vi "Client CR.vi"() -> ()   [LabVIEW 2021]
uses:
  Master CR/Examples/PM3112/enums/main_prog_state.ctl
  Master CR/Examples/PM3112/enums/init_state.ctl
  WebSockets/WebSocket Client CR/WebSocket Client CR.lvclass
  Master CR/Param/TCP Param/TCP Param.lvclass
  D:/my_projects/projects/Algorithms/Labview/21/Master CR/Param/Param.lvclass
  WebSockets/WebSocket Client CR/WebSocket Client CR.lvclass/WebSocket Client CR.ctl
  Master CR/Param/Param.lvclass/Param.ctl
  Master CR/Param/TCP Param/TCP Param.lvclass/TCP Param.ctl
  <vilib>/Platform/TimedLoop/XDataNode/timing_clust.ctl
  <vilib>/Platform/TimedLoop/XDataNode/nitl_modes.ctl
  <vilib>/Platform/TimedLoop/XDataNode/wakeup.ctl
  Master CR/Examples/PM3112/enums/close_state.ctl
  <vilib>/Platform/TimedLoop/XDataNode/XDataNode.xnode
  Modbus_v121c/Data Model/Device Data Model.lvclass
  <vilib>/Platform/TimedLoop/XDataNode/XDNodeRunTimeDep.lvlib
  Master CR/Examples/PM3112/enums/Param_MB test.lvlib
  Master CR/Param/Param.lvclass
panel:
  in  "Send String Data":string[](array[string])
  out "String Data":string[](array[string])
  in  "Write":bool
  in  "Read":bool
  out "connects":bool[](array[boolean])
  out "Binary Data":u8[][](array[numeric])
  in  "Send Binary Data":u16[][](array[numeric])
  out "comm error":errorcluster
  out "initialise error":errorcluster
  in  "EP_on":bool
  in  "tick":i64=100 caption="Время цикла основной программы" min=5 max=500 step=1
  in  "stop":bool
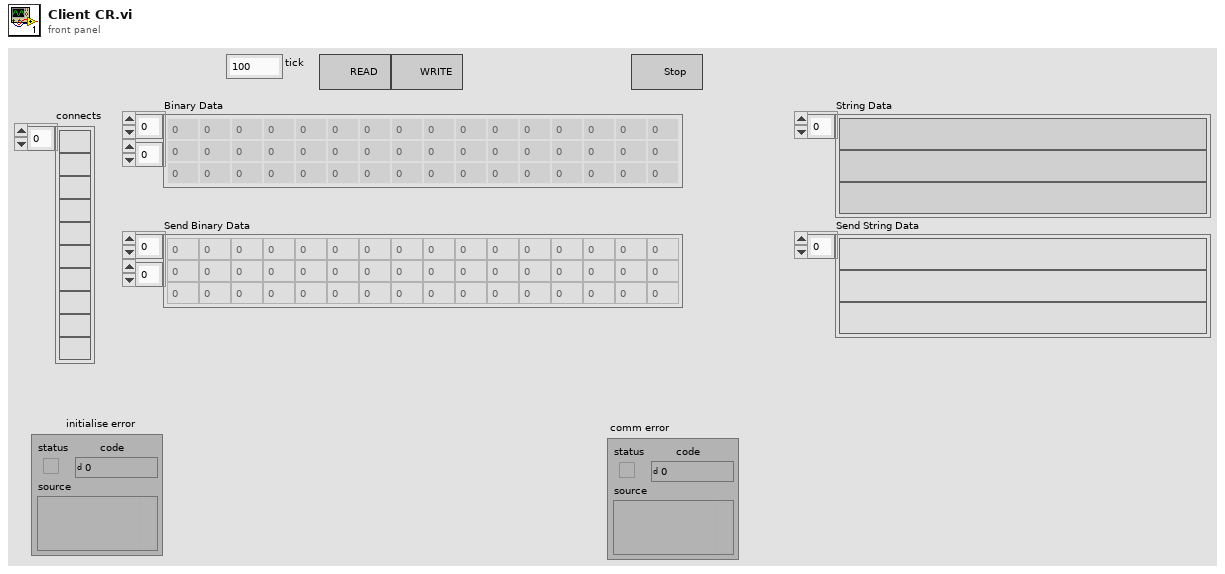
[diagram p1: front panel]
types:
  T1 = cluster{"conn_timeout":i32, "reconn_timeout":i32, "N attempt max":i32, "t_reset_TTL":i32, "write_timeout":i32, "read_timeout":i32, "period":i32}[]
  T2 = cluster{"Remote IP Address":string, "Remote Port":u16}[]
  T3 = typedef "Param_MB test.lvlib/init_state.ctl" = enum16{"Init Data", "Init TMPs", "Init system DB", "Init data DB", "Read Enums", "Init arrays", "Init KFM", "Init Param", "Init AI param", "Init DI param", "Init AO param", "Init DO param", "Init ALR param", "Init save progs", "Read OPC param", "Init Shared Variables", "Init regulators", "Init heaters", "Init Y defs", "Exit"}
  T4 = typedef "Param_MB test.lvlib/main_prog_state.ctl" = enum16{"Read_AI_Param", "Read_DI_Param", "Read_AO_Param", "Read_DO_Param", "Read_ALR_ON_OFF", "Read_ALR_Param", "Read_Param", "Read_REG_Param", "Timers", "AI", "DI", "SendAItoScada", "SendDItoScada", "Alarms", "SendAItoDB", "SendDItoDB", "SendALRtoDB", "Messages", "Controls", "Control HT1", "QN_control", "QN", "QN_state", "Control EB3", "Outputs", "Exit"}
  T5 = cluster{"KFM":string[], "PAR":string[], "AI":string[], "DI":string[], "DI_fast":string[], "AO":string[], "Regs":string[], "DO":string[], "ALR":string[], "System":string[]}
  T6 = cluster{"Enums":cluster{"KFM":string[], "PAR":string[], "AI":string[], "DI":string[], "DI_fast":string[], "AO":string[], "Regs":string[], "DO":string[], "ALR":string[], "System":string[]}, "WSs":refnum<class "WebSocket Client CR.lvclass">[]}
  T7 = cluster{"current time":timestamp, "Timer_1s":bool, "Timer_10s":bool, "Timer_1day":bool}
  T8 = typedef "XDNodeRunTimeDep.lvlib/timing_clust.ctl" = cluster{"Expected End [f-1]":u64, "Actual End [f-1]":u64, "Finished Late? [f-1]":bool, "Expected End [i-1]":u64, "Actual End [i-1]":u64, "Finished Late? [i-1]":bool, "Expected Start [i]":u64, "Actual Start [i]":u64, "Expected Start [f]":u64, "Actual Start [f]":u64, "Source Name":string, "Structure Name":string, "Period":i64, "Deadline":i64, "Offset":i64, "Start":i64, "Priority":i32, "Timeout":i32, "Mode":T9, "Wakeup Reason":T10, "Error":errorcluster, "Source Type":string, "Secondary Source Type":string, "Global End Time":u64, "Global Start Time":u64, "Frame Duration":u64, "Iteration Duration":u64, "Assigned CPU":i32, "I/O Scan Engine Mode":u32}
  T9 = typedef "XDNodeRunTimeDep.lvlib/nitl_modes.ctl" = enum32{"No Change", "Process missed periods, maintain original phase", "Discard missed periods, maintain original phase", "Process missed periods, ignore original phase", "Discard missed periods, ignore original phase"}
  T10 = typedef "XDNodeRunTimeDep.lvlib/wakeup.ctl" = enum32{"Normal", "Aborted", "Asynchronous wakeup", "Timing source error", "Timed loop error", "Timeout"}
  T11 = typedef "Param_MB test.lvlib/close_state.ctl" = enum16{"QN_state notifier", "QN_control_queue", "ALR notifires", "ALR", "DO notifires", "DO", "AO notifires", "AO", "DI notifres", "DI", "AI notifires", "AI", "OPC", "Param", "SaveMessageProg", "KFM DadaRef", "KFM Registers", "KFM StatusRef", "Exit"}
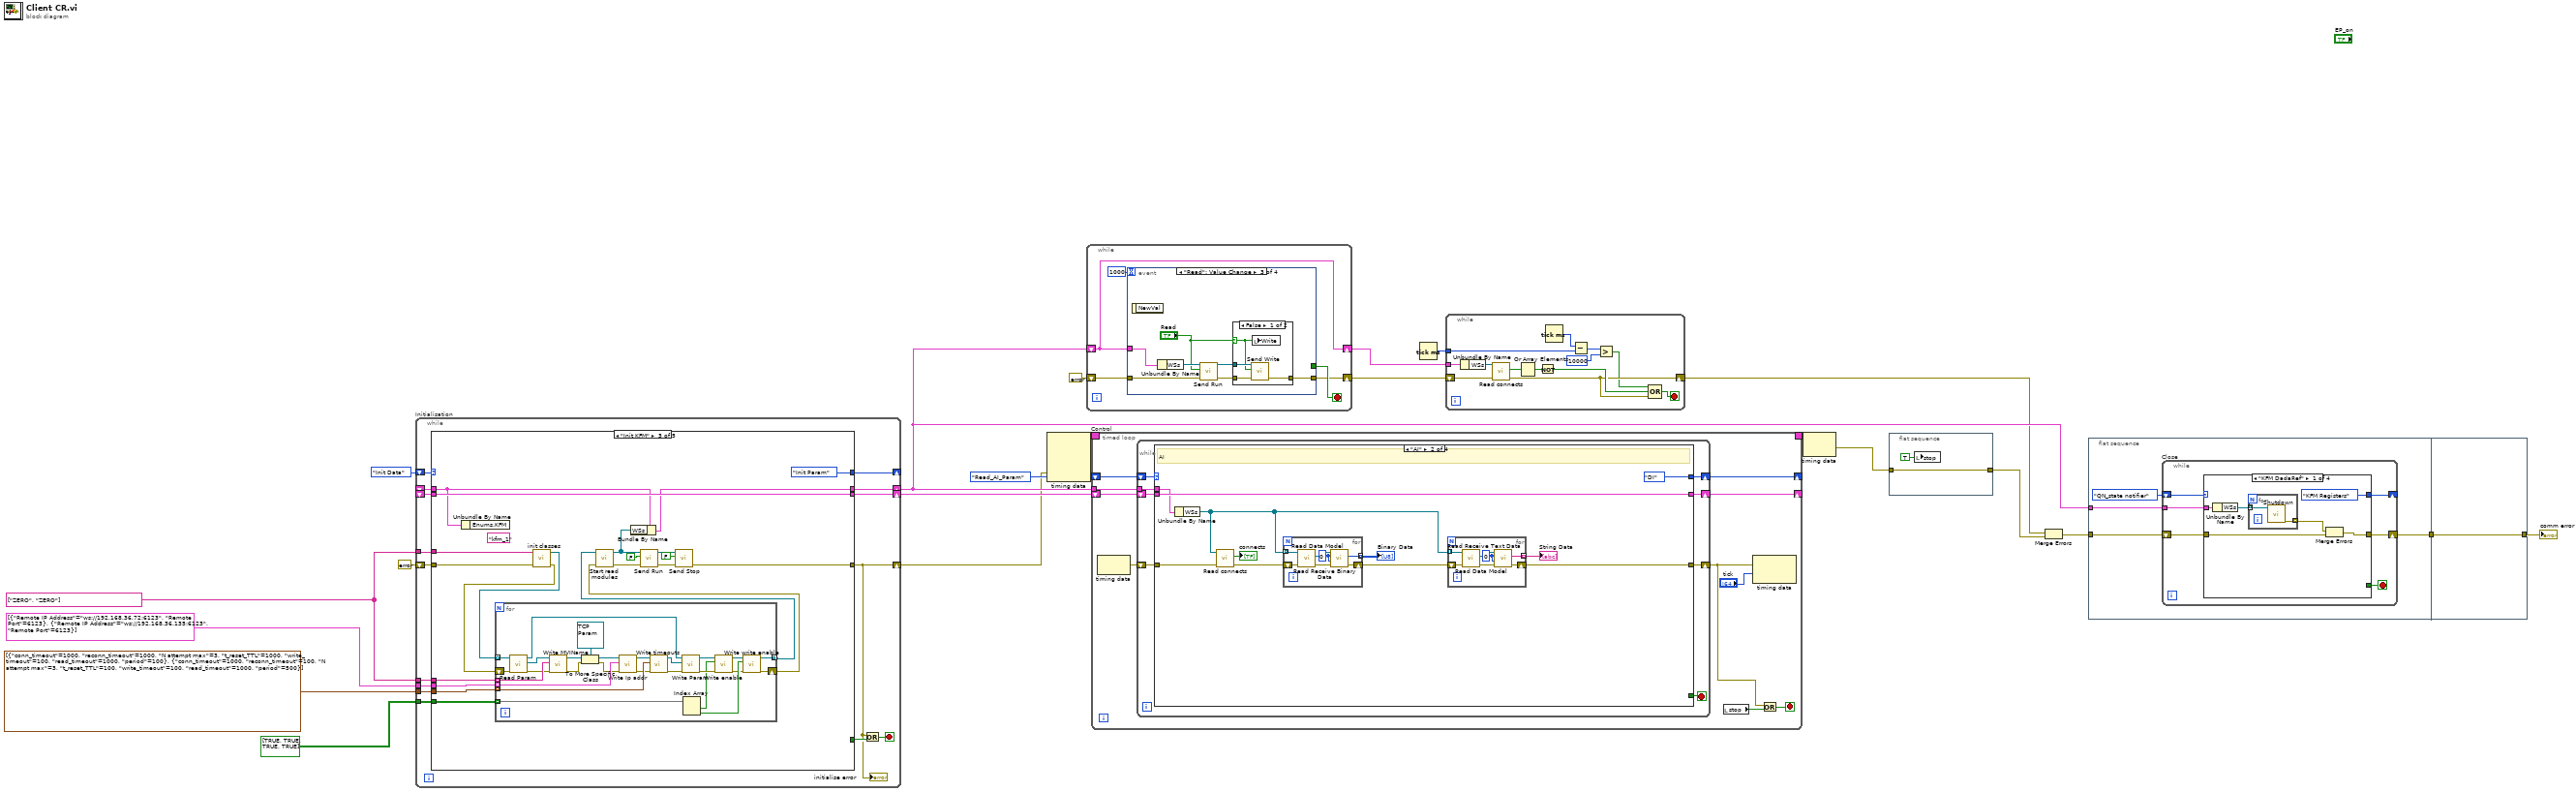
[diagram p0: block diagram]
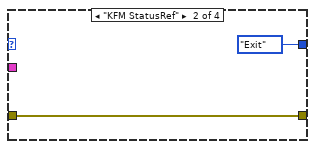
[diagram p2: hidden frame]
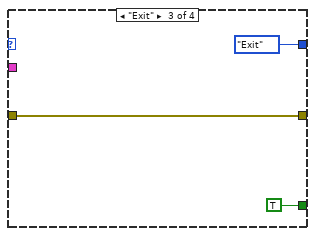
[diagram p3: hidden frame]
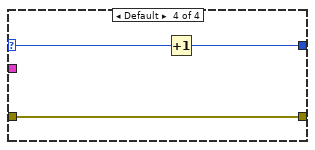
[diagram p4: hidden frame]
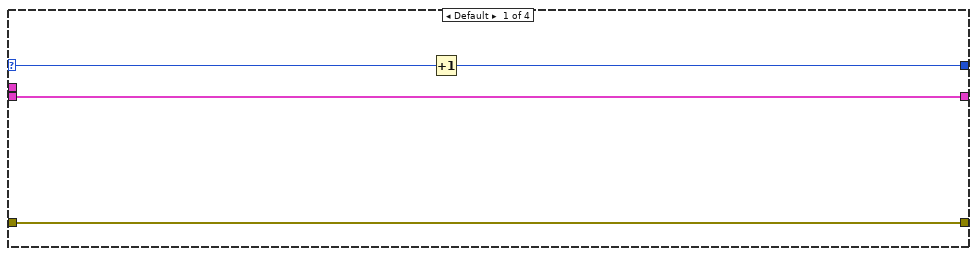
[diagram p5: hidden frame]
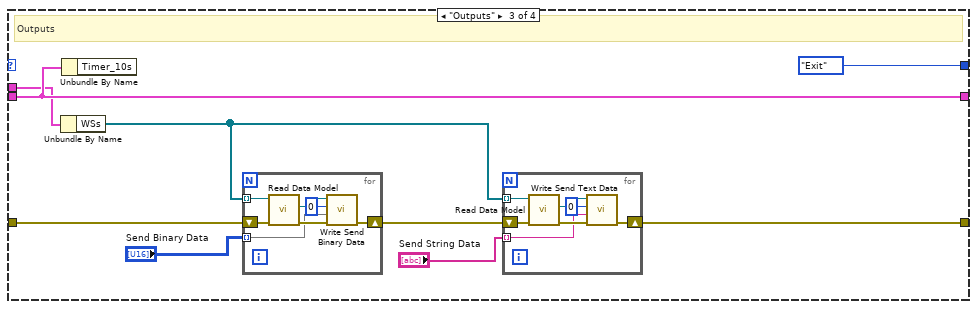
[diagram p6: hidden frame]
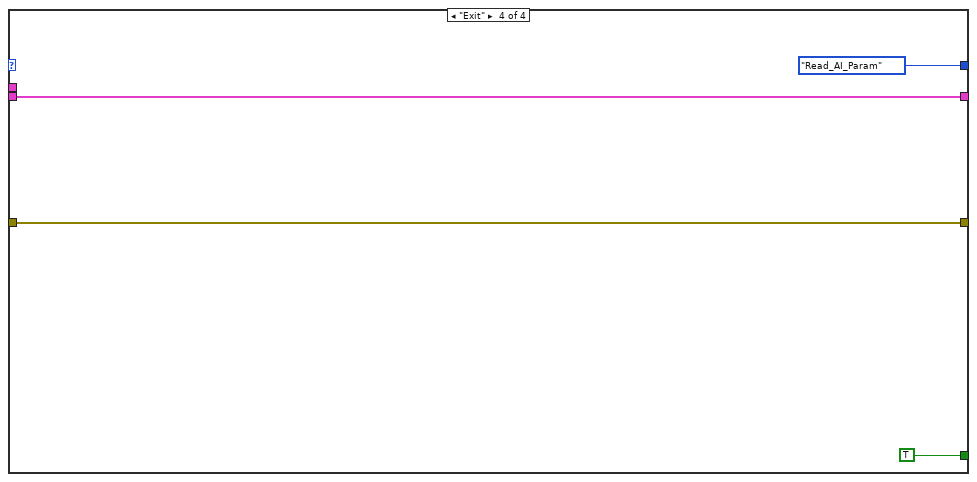
[diagram p7: hidden frame]
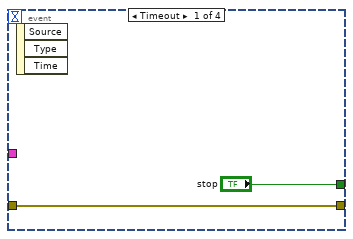
[diagram p8: hidden frame]
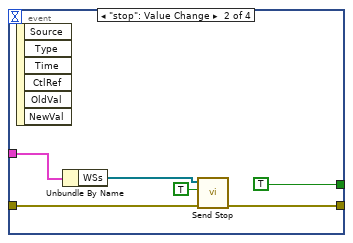
[diagram p9: hidden frame]
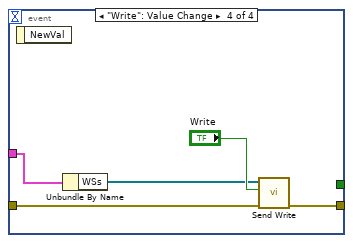
[diagram p11: hidden frame]
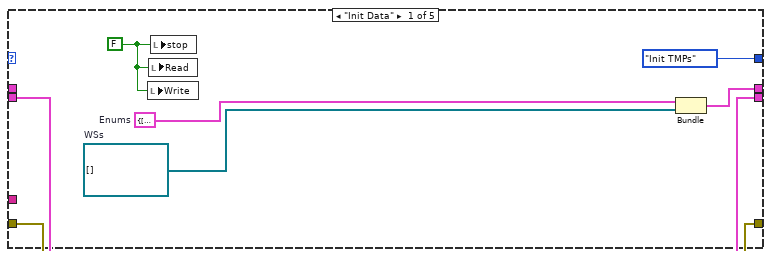
[diagram p12: hidden frame]
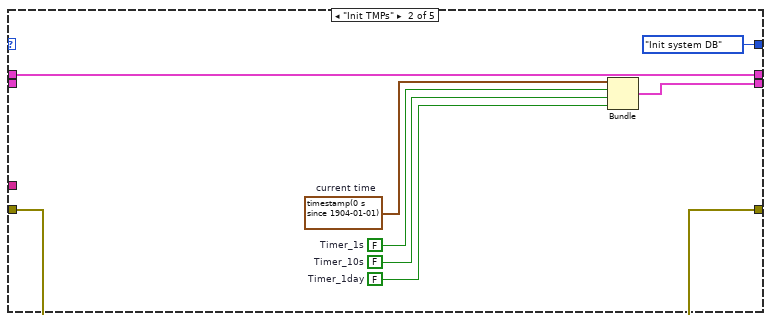
[diagram p13: hidden frame]
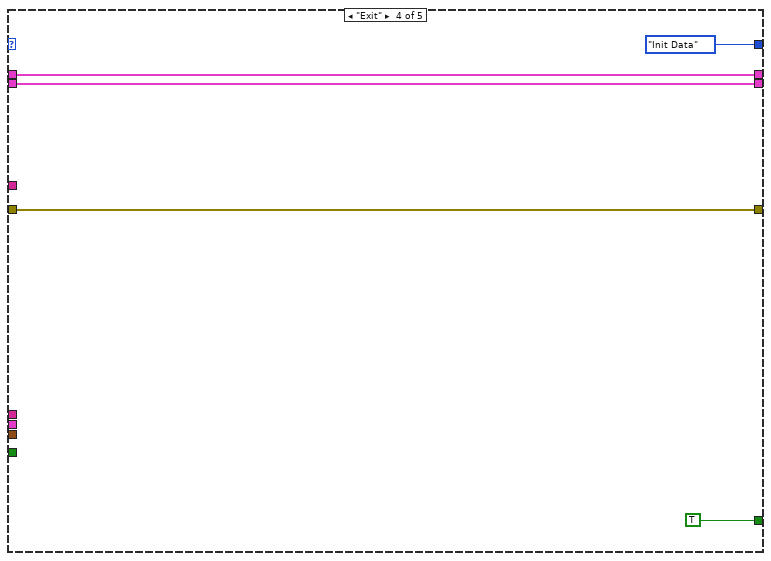
[diagram p14: hidden frame]
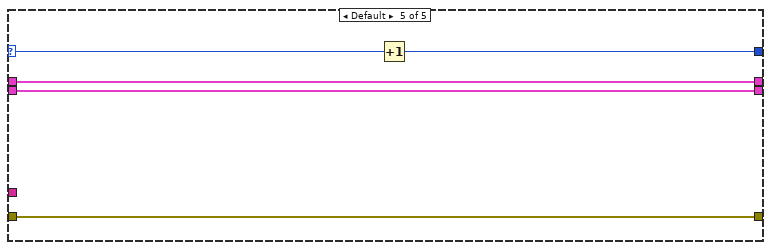
[diagram p15: hidden frame]
diagram:
  w8 = string[] ["ZERO", "ZERO"] ("MVIName")
  n1 = while "Initialisation" {
    shift-right: [w28] -> w7
    shift-left: errorcluster {"status"=FALSE, "code"=0, "source"=""} ("error out") -> [w34]
    shift-right: [w37] -> w13
    shift-left: _ -> [w35]
    shift-right: [w33] -> _
    shift-left: init_state."Init Data" -> [w36]
    shift-right: [w30] -> w16
    shift-left: _ -> [w29]
    tunnel: w8 -> [w27]
    tunnel: T2 [{"Remote IP Address"="ws://192.168.36.72:6123", "Remote Port"=6123}, {"Remote IP Address"="ws://192.168.36.135:6123", "Remote Port"=6123}] ("IP Address") -> [w26]
    tunnel: T1 [{"conn_timeout"=1000, "reconn_timeout"=1000, "N attempt max"=3, "t_reset_TTL"=1000, "write_timeout"=100, "read_timeout"=1000, "period"=100}, {"conn_timeout"=1000, "reconn_timeout"=100, "N attempt max"=3, "t_reset_TTL"=100, "write_timeout"=100, "read_timeout"=1000, "period"=500}] ("timeouts") -> [w25]
    tunnel: bool[][] [[TRUE, TRUE], [TRUE, TRUE]] ("enable") -> [w24]
    tunnel: w8 -> [w23]
    stop <- w31 stop-if-true
    # "Initialisation"
    n2 = case shown="\"Init KFM\"" w36 {
      tunnel: [w42 w51 w53 w102 w105] -> w28
      selector: w36 -> [_ _ _ _ w108]
      tunnel: [w43 w50 w54 w103 w106] -> w37
      tunnel: w35 -> [_ w50 w71 w103 w106]
      tunnel: w34 -> [w42 w51 w70 w102 w105]
      tunnel: [init_state."Init TMPs" init_state."Init system DB" init_state."Init Param" init_state."Init Data" w107] -> w33
      tunnel: [_ _ _ TRUE _] -> w32
      tunnel: [w40 w49 w72 w100 w109] -> w30
      tunnel: w29 -> [w40 _ w72 w100 w109]
      tunnel: w27 -> [_ _ w65 _ _]
      tunnel: w26 -> [_ _ w64 _ _]
      tunnel: w25 -> [_ _ w63 _ _]
      tunnel: w24 -> [_ _ w62 _ _]
      tunnel: w23 -> [_ _ w61 _ _]
      frame "Init Data" {
        w38 = refnum<class "WebSocket Client CR.lvclass">[] []  # WSs
        w39 = FALSE ("stop")
        w41 = T5 {"KFM"=[], "PAR"=[], "AI"=[], "DI"=[], "DI_fast"=[], "AO"=[], "Regs"=[], "DO"=[], "ALR"=[], "System"=[]}  # Enums
        n3 = local write "Write"(w39) -> ()
        n4 = local write "Read"(w39) -> ()
        n5 = local write "stop"(w39) -> ()
        n6 = Bundle("Enums"=w41, "WSs"=w38) -> (w43:T6)  [unwired: 1 in]
      }
      frame "Init TMPs" {
        w45 = FALSE  # Timer_10s
        w46 = FALSE  # Timer_1day
        w47 = FALSE  # Timer_1s
        w48 = timestamp(0 s since 1904-01-01)  # current time
        n7 = Bundle("current time"=w48, "Timer_1s"=w47, "Timer_10s"=w45, "Timer_1day"=w46) -> (w49:T7)  [unwired: 1 in]
      }
      frame "Init KFM" {
        (unwired) "kfm_1" ("KFMTable")
        n8 = Unbundle By Name(w71) -> ()  [unwired: 1 out]
        n9 = call "init classes.vi"("error in (no error)"=w70, "MVINames"=w61) -> ("error out"=w67:errorcluster, "MBs"=w69:refnum<class "WebSocket Client CR.lvclass">[])  [unwired: 8 in]
        n10 = for {
          tunnel: w69 -> [w75] mode=indexing
          tunnel: w64 -> [w82] mode=indexing
          tunnel: w63 -> [w79] mode=indexing
          tunnel: w65 -> [w97] mode=indexing
          tunnel: w62 -> [w91] mode=indexing
          tunnel: [w87] -> w68 mode=indexing
          shift-right: [w86] -> w66
          shift-left: w67 -> [w99]
          n11 = call "Read Param.vi"("error in (no error)"=w99, "MB_TCP in"=w75) -> ("error out"=w95:errorcluster, "Param"=w74:refnum<class "Param.lvclass">, "MB_TCP out"=w94:refnum<class "WebSocket Client CR.lvclass">)  [unwired: 7 in]
          n12 = call "Write MVIName.vi"("error in (no error)"=w95, "MVIName"=w97, "MB Param in"=w74) -> ("error out"=w84:errorcluster, "MB Param out"=w96:refnum<class "Param.lvclass">)  [unwired: 7 in]
          n13 = To More Specific Class(target class=refnum<class "TCP Param.lvclass"> refnum ("Param.lvlib:TCP Param.lvclass"), reference=w96, error in=w84) -> (specific class reference=w83:refnum<class "TCP Param.lvclass">, error out=w81:errorcluster)
          n14 = call "Write Ip addr.vi"("error in (no error)"=w81, "IP address"=w82, "MB Param in"=w83) -> ("error out"=w78:errorcluster, "MB Param out"=w80:refnum<class "TCP Param.lvclass">)  [unwired: 7 in]
          n15 = call "Write timeouts.vi"("error in (no error)"=w78, "timeouts"=w79, "MB Param in"=w80) -> ("error out"=w77:errorcluster, "MB Param out"=w76:refnum<class "TCP Param.lvclass">)  [unwired: 7 in]
          n16 = call "Write Param.vi"("error in (no error)"=w77, "Param"=w76, "MB_TCP in"=w94) -> ("error out"=w92:errorcluster, "MB_TCP out"=w93:refnum<class "WebSocket Client CR.lvclass">)  [unwired: 7 in]
          n17 = Index Array(array=w91) -> (element #1=w90:bool, element #2=w89:bool)  [unwired: 2 in]
          n18 = call "Write enable.vi"("error in (no error)"=w92, "enable"=w90, "Master CR in"=w93) -> ("error out"=w88:errorcluster, "Master CR out"=w98:refnum<class "WebSocket Client CR.lvclass">)  [unwired: 7 in]
          n19 = call "Write write enable.vi"("error in (no error)"=w88, "write enable"=w89, "Master CR in"=w98) -> ("error out"=w86:errorcluster, "Master CR out"=w87:refnum<class "WebSocket Client CR.lvclass">)  [unwired: 7 in]
        }
        n20 = call "Start read modules.vi"("error in"=w66, "classes"=w68) -> ("error out"=w56:errorcluster, "classes initialised"=w55:refnum<class "WebSocket Client CR.lvclass">[])  [unwired: 8 in]
        n21 = Bundle By Name(cluster=w71, "WSs"=w55) -> (w54:T6)
        n22 = call "Send Run.vi"("error in"=w56, "Run"=FALSE, "MCRs"=w55) -> ("error out"=w59:errorcluster, "MCRs out"=w60:refnum<class "WebSocket Client CR.lvclass">[])  [unwired: 7 in]
        n23 = call "Send Stop.vi"("error in"=w59, "Stop"=FALSE ("Write"), "MCRs"=w60) -> ("error out"=w53:errorcluster)  [unwired: 7 in, 1 out]
      }
      frame "Exit" {
      }
      frame Default {
        n24 = Increment(x=w108) -> (x+1=w107:T3)
      }
    }
    "initialise error" <- w28
    n25 = Or(x=w28, y=w32) -> (x .or. y?=w31:bool)
  }
  n26 = node-c288(w7) -> (w22:T8)  [unwired: 3 in]
  n27 = while {
    shift-right: [w112] -> w4
    shift-left: errorcluster {"status"=FALSE, "code"=0, "source"=""} ("error out") -> [w111]
    shift-right: [w110] -> w3
    shift-left: w13 -> [w110]
    stop <- w113 stop-if-true
    n28 = event shown="[2] \"Read\": Value Change" {
      selector: _ -> [_ _ _ _]
      dyn-events: _ -> [_ _ _ _]
      timeout: 1000 -> [_ _ _ _]
      tunnel: ["stop" TRUE ("stop") _ _] -> w113
      tunnel: w110 -> [_ w117 w129 w139]
      tunnel: w111 -> [w115 w121 w128 w138]
      tunnel: [w115 w120 w123 w137] -> w112
      event Timeout {
        n29 = event-data() -> ()  [unwired: 1 in, 3 out]
      }
      event "stop": Value Change {
        n30 = event-data() -> ()  [unwired: 1 in, 6 out]
        n31 = Unbundle By Name(w117) -> ("WSs"=w118:refnum<class "WebSocket Client CR.lvclass">[])
        n32 = call "Send Stop.vi"("error in"=w121, "Stop"=TRUE, "MCRs"=w118) -> ("error out"=w120:errorcluster)  [unwired: 7 in, 1 out]
      }
      event "Read": Value Change {
        n33 = event-data() -> ()  [unwired: 1 in, 1 out]
        n34 = Unbundle By Name(w129) -> ("WSs"=w127:refnum<class "WebSocket Client CR.lvclass">[])
        n35 = call "Send Run.vi"("error in"=w128, "Run"="Read", "MCRs"=w127) -> ("error out"=w125:errorcluster, "MCRs out"=w124:refnum<class "WebSocket Client CR.lvclass">[])  [unwired: 7 in]
        n36 = case shown="False" "Read" {
          selector: "Read" -> [w131 _]
          tunnel: w125 -> [w133 w134]
          tunnel: w124 -> [w132 _]
          tunnel: [w130 w134] -> w123
          frame False {
            n37 = call "Send Write.vi"("error in"=w133, "Write"=w131, "MCRs"=w132) -> ("error out"=w130:errorcluster)  [unwired: 7 in, 1 out]
            n38 = local write "Write"(w131) -> ()
          }
          frame True {
          }
        }
      }
      event "Write": Value Change {
        n39 = event-data() -> ()  [unwired: 1 in, 1 out]
        n40 = Unbundle By Name(w139) -> ("WSs"=w135:refnum<class "WebSocket Client CR.lvclass">[])
        n41 = call "Send Write.vi"("error in"=w138, "Write"="Write", "MCRs"=w135) -> ("error out"=w137:errorcluster)  [unwired: 7 in, 1 out]
      }
    }
  }
  n42 = timed-loop "Control" {
    tunnel: w13 -> [w149]
    shift-right: [w147] -> _
    shift-left: w16 -> [w148]
    timing: w22 -> [_]
    timing-out: [_] -> w21
    shift-right: [w145] -> _
    shift-left: main_prog_state."Read_AI_Param" -> [w144]
    stop <- w142 stop-if-true
    n43 = node-c288() -> (w146:errorcluster)  [unwired: 1 in]
    n44 = while {
      tunnel: w149 -> [w157]
      shift-right: [w155] -> w147
      shift-left: w148 -> [w156]
      shift-right: [w150] -> w140
      shift-left: w146 -> [w154]
      shift-right: [w153] -> w145
      shift-left: w144 -> [w152]
      stop <- w151 stop-if-true
      n45 = case shown="\"AI\"" w152 {
        tunnel: w154 -> [w158 w171 w191 w210]
        tunnel: w157 -> [_ w167 w193 _]
        tunnel: w156 -> [w160 w170 w194 w211]
        tunnel: [w160 w170 w194 w211] -> w155
        selector: w152 -> [w161 _ _ _]
        tunnel: [w159 main_prog_state."DI" main_prog_state."Exit" main_prog_state."Read_AI_Param"] -> w153
        tunnel: [_ _ _ TRUE] -> w151
        tunnel: [w158 w162 w189 w210] -> w150
        frame Default {
          n46 = Increment(x=w161) -> (x+1=w159:T4)
        }
        frame "AI" {
          # "AI"
          n47 = Unbundle By Name(w167) -> ("WSs"=w164:refnum<class "WebSocket Client CR.lvclass">[])
          n48 = call "Read connects.vi"("error in (no error)"=w171, "MCRs in"=w164) -> ("error out"=w168:errorcluster, "connects"=→"connects":bool[])  [unwired: 7 in, 1 out]
          n49 = for {
            tunnel: w164 -> [w183] mode=indexing
            shift-right: [w186] -> w165
            shift-left: w168 -> [w184]
            tunnel: [w185] -> w166 mode=indexing
            w180 = u16 0 ("starting address")
            n50 = call "Read Data Model.vi"("error in (no error)"=w184, "Master CR in"=w183) -> ("error out"=w182:errorcluster, "Data Model"=w181:refnum<class "Device Data Model.lvclass">)  [unwired: 7 in, 1 out]
            n51 = call-dynamic "Read Receive Binary Data.vi"("error in (no error)"=w182, "number of registers"=w180, "starting address"=w180, "device data model in"=w181) -> ("error out"=w186:errorcluster, "data"=w185:u8[])  [unwired: 5 in, 1 out]
          }
          "Binary Data" <- w166
          n52 = for {
            tunnel: w164 -> [w177] mode=indexing
            shift-right: [w179] -> w162
            shift-left: w165 -> [w178]
            tunnel: [w174] -> w163 mode=indexing
            w173 = u16 0 ("starting address")
            n53 = call "Read Data Model.vi"("error in (no error)"=w178, "Master CR in"=w177) -> ("error out"=w176:errorcluster, "Data Model"=w175:refnum<class "Device Data Model.lvclass">)  [unwired: 7 in, 1 out]
            n54 = call-dynamic "Read Receive Text Data.vi"("error in (no error)"=w176, "number of registers"=w173, "starting address"=w173, "device data model in"=w175) -> ("error out"=w179:errorcluster, "data"=w174:string)  [unwired: 5 in, 1 out]
          }
          "String Data" <- w163
        }
        frame "Outputs" {
          # "Outputs"
          n55 = Unbundle By Name(w193) -> ("WSs"=w188:refnum<class "WebSocket Client CR.lvclass">[])
          n56 = Unbundle By Name(w194) -> ()  [unwired: 1 out]
          n57 = for {
            tunnel: w188 -> [w207] mode=indexing
            shift-right: [w209] -> w190
            shift-left: w191 -> [w208]
            tunnel: "Send Binary Data" -> [w204] mode=indexing
            n58 = call "Read Data Model.vi"("error in (no error)"=w208, "Master CR in"=w207) -> ("error out"=w206:errorcluster, "Data Model"=w205:refnum<class "Device Data Model.lvclass">)  [unwired: 7 in, 1 out]
            n59 = call-dynamic "Write Send Binary Data.vi"("error in (no error)"=w206, "values"=w204, "starting address"=u16 0, "standard data model in"=w205) -> ("error out"=w209:errorcluster)  [unwired: 6 in, 1 out]
          }
          n60 = for {
            tunnel: w188 -> [w200] mode=indexing
            shift-right: [w202] -> w189
            shift-left: w190 -> [w201]
            tunnel: "Send String Data" -> [w197] mode=indexing
            n61 = call "Read Data Model.vi"("error in (no error)"=w201, "Master CR in"=w200) -> ("error out"=w199:errorcluster, "Data Model"=w198:refnum<class "Device Data Model.lvclass">)  [unwired: 7 in, 1 out]
            n62 = call-dynamic "Write Send Text Data.vi"("error in (no error)"=w199, "values"=w197, "starting address"=u16 0, "standard data model in"=w198) -> ("error out"=w202:errorcluster)  [unwired: 6 in, 1 out]
          }
        }
        frame "Exit" {
        }
      }
    }
    n63 = local read "stop"() -> (w141:bool)
    n64 = node-c288(w140, "tick") -> ()  [unwired: 1 out]
    n65 = Or(x=w140, y=w141) -> (x .or. y?=w142:bool)
  }
  n66 = Tick Count (ms)() -> (millisecond timer value=w2:u32)
  n67 = while {
    shift-right: [w225] -> w1
    shift-left: w4 -> [w232]
    tunnel: w3 -> [w229]
    tunnel: w2 -> [w223]
    stop <- w227 stop-if-true
    n68 = Unbundle By Name(w229) -> ("WSs"=w228:refnum<class "WebSocket Client CR.lvclass">[])
    n69 = call "Read connects.vi"("error in (no error)"=w232, "MCRs in"=w228) -> ("error out"=w225:errorcluster, "connects"=w231:bool[])  [unwired: 7 in, 1 out]
    n70 = Or Array Elements(Boolean array=w231) -> (logical OR=w230:bool)
    n71 = Not(x=w230) -> (.not. x?=w226:bool)
    n72 = Tick Count (ms)() -> (millisecond timer value=w224:u32)
    n73 = Subtract(x=w224, y=w223) -> (x-y=w222:u32)
    n74 = Greater?(x=w222, y=u32 10000) -> (0:w220:bool)
    n75 = Compound Arithmetic op=OR(w220, w226, w225) -> (w227:bool)
  }
  n76 = node-c288(w21) -> (w6:errorcluster)
  n77 = flat-sequence {
    tunnel: [w233] -> w5
    tunnel: w6 -> [w233]
    frame #0 {
      n78 = local write "stop"(TRUE ("stop")) -> ()
    }
  }
  n79 = Merge Errors(w1, w5) -> (w15:errorcluster)
  n80 = flat-sequence {
    tunnel: w13 -> [w237]
    tunnel: w15 -> [w236]
    tunnel: [w235] -> w14
    tunnel: [w261] -> w19
    tunnel: w14 -> [w261]
    frame #0 {
      n81 = while "Close" {
        shift-right: [w243] -> _
        shift-left: close_state."QN_state notifier" ("Init_state") -> [w244]
        tunnel: w237 -> [w241]
        shift-right: [w239] -> w235
        shift-left: w236 -> [w240]
        stop <- w242 stop-if-true
        n82 = case shown="\"KFM DadaRef\"" w244 {
          selector: w244 -> [_ _ _ w260]
          tunnel: [close_state."KFM Registers" close_state."Exit" close_state."Exit" w259] -> w243
          tunnel: [_ _ TRUE _] -> w242
          tunnel: w241 -> [w250 _ _ _]
          tunnel: w240 -> [w248 w253 w256 w258]
          tunnel: [w247 w253 w256 w258] -> w239
          frame "KFM DadaRef" {
            n83 = Unbundle By Name(w250) -> ("WSs"=w246:refnum<class "WebSocket Client CR.lvclass">[])
            n84 = for {
              tunnel: w246 -> [w252] mode=indexing
              tunnel: [w251] -> w245 mode=indexing
              n85 = call-dynamic "Shutdown.vi"("WS in"=w252) -> ("error out"=w251:errorcluster)  [unwired: 10 in]
            }
            n86 = Merge Errors(w245, w248) -> (w247:errorcluster)
          }
          frame "KFM StatusRef" {
          }
          frame "Exit" {
          }
          frame Default {
            n87 = Increment(x=w260) -> (x+1=w259:T11)
          }
        }
      }
    }
    frame #1 {
    }
  }
  "comm error" <- w19
